vi "chaos crest cu get key value.vi"(6 "maxsize":i32, 7 "values":string, 9 "keys":string, 10 "cuname":string, 11 "handleConnection":u32) -> (1 "keys out":string, 2 "timestamp":u64, 3 "handleConnection out":u32, 5 "values out":string)   [LabVIEW 2014, in "libcommon-crest.lvlib"]
doc: "uint64_t chaos_crest_cu_get_key_value(chaos_crest_handle_t h,const char*cuname,char*keys,char*values,int maxsize);"
uses:
  libcommon-crest.lvlib
  chaos-i686-dynamic-release/lib/libcommon-crest.so
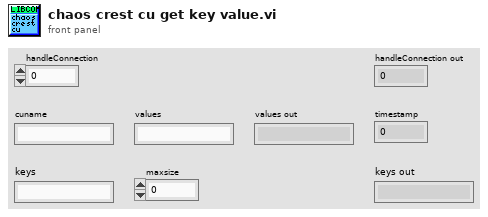
[diagram p1: front panel]
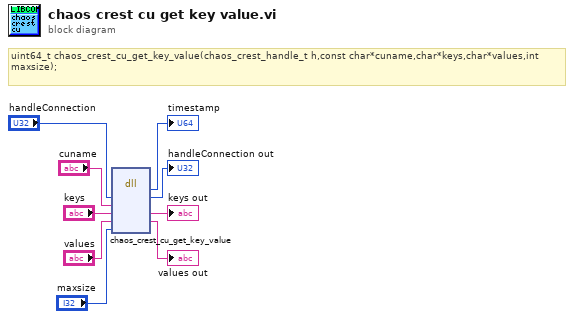
[diagram p0: block diagram]
diagram:
  # "uint64_t chaos_crest_cu_get_key_value(chaos_crest_handle_t h,const char*cuname,char*keys,char*values,int maxsize);"
  n1 = dll-call lib="home/chaos/chaos_bundle/chaos-i686-dynamic-release/lib/libcommon-crest.*" fn="chaos_crest_cu_get_key_value"("handleConnection"="handleConnection", "cuname"="cuname", "keys"="keys", "values"="values", "maxsize"="maxsize") -> ("return type"=→"timestamp":u64, "handleConnection"=→"handleConnection out":u32, "keys"=→"keys out":string, "values"=→"values out":string)  [unwired: 5 in, 2 out]
